vi "Parse Params-JSONtext.vi"(8 "error in (no error)":errorcluster, 10 "JSON":string) -> (0 "error out":errorcluster, 1 "Params":string[](array[string]), 2 "Names":string[](array[string]))   [LabVIEW 2019, in "JSON-RPC.lvclass"]
uses:
  JSON-RPC.lvclass
  <vilib>/JDP Science/JSONtext/JSONtext.lvlib
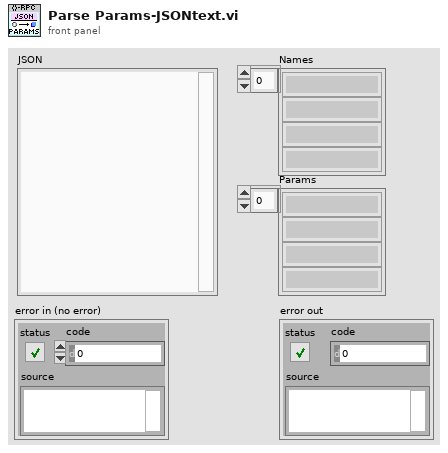
[diagram p1: front panel]
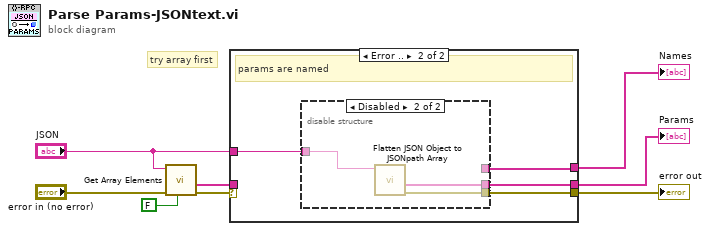
[diagram p0: block diagram]
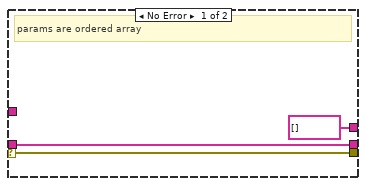
[diagram p2: hidden frame]
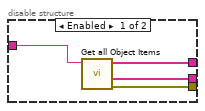
[diagram p3: hidden frame]
diagram:
  # "try array first"
  n1 = call <vilib>:"Get Array Elements.vi"("Pass non-arrays"=FALSE, "error in (no error)"="error in (no error)", "JSON"="JSON") -> ("error out"=w8:errorcluster, "<JSON>"=w7:string[])  [unwired: 6 in, 1 out]
  n2 = case shown="Error .." w8 {
    selector: w8 -> [w10 _]
    tunnel: [w11 w14] -> w2
    tunnel: w7 -> [w11 _]
    tunnel: [w10 w13] -> w3
    tunnel: "JSON" -> [_ w15]
    tunnel: [string[] [] ("Item Names") w12] -> w1
    frame No Error {
      # "params are ordered array"
    }
    frame Error {
      # "params are named"
      n3 = disable-structure shown="Disabled" {
        disable-tunnel: w15 -> [w16 w22]
        disable-tunnel: [w19 w21] -> w14
        disable-tunnel: [w18 w20] -> w13
        disable-tunnel: [w17 _] -> w12
        frame Enabled {
          n4 = call <vilib>:"Get all Object Items.vi"("JSON"=w16) -> ("error out"=w18:errorcluster, "<JSON>"=w19:string[], "Item Names"=w17:string[])  [unwired: 7 in, 1 out]
        }
        frame Disabled {
          n5 = call <vilib>:"Flatten JSON Object to JSONpath Array.vi"("JSON"=w22) -> ("error out"=w20:errorcluster, "<JSON>"=w21:string[])  [unwired: 8 in, 1 out]
        }
      }
    }
  }
  "error out" <- w3
  "Params" <- w2
  "Names" <- w1
